vi "WidgetLocation.vi"(6 "error in":errorcluster, 9 "Array in":refnum<class "Array.lvclass">) -> (0 "error out":errorcluster, 3 "Array out":refnum<class "Array.lvclass">, 4 "Bounds":T1, 5 "Location":T2)   [LabVIEW 2014, in "Raspberry Pi Compatible Compiler for LabVIEW.lvlib" / "Array.lvclass"]
uses:
  Array.lvclass
  <vilib>/Utility/miscctls.llb/LVPositionTypeDef.ctl
  <vilib>/Utility/miscctls.llb/LVBoundsTypeDef.ctl
  Control/Control.lvclass
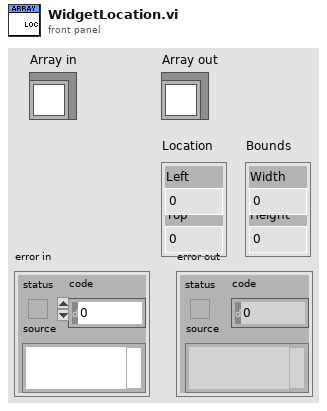
[diagram p1: front panel]
types:
  T1 = typedef "LVBoundsTypeDef.ctl" = cluster{"Width":u32, "Height":u32}
  T2 = typedef "LVPositionTypeDef.ctl" = cluster{"Left":i32, "Top":i32}
  T3 = typedef "LVRectTypeDef.ctl" = cluster{"Left":i16, "Top":i16, "Right":i16, "Bottom":i16}
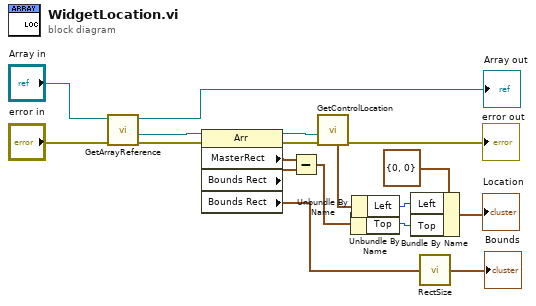
[diagram p0: block diagram]
diagram:
  n1 = call "GetArrayReference.vi"("error in"="error in", "Array in"="Array in") -> ("error out"=w15:errorcluster, "array reference"=w16:refnum<vi>, "Array out"=→"Array out":refnum<class "Array.lvclass">)  [unwired: 7 in]
  n2 = property class="Arr"(reference=w16, error in=w15) -> (reference out=w4:refnum<vi>, error out=w5:errorcluster, "MasterRect"=w14:T3, "Bounds Rect"=w13:T3, "Bounds Rect"=w12:T3)
  n3 = Subtract(x=w14, y=w13) -> (x-y=w8:T3)
  n4 = call "GetControlLocation.vi"("error in"=w5, "Control in"=w4) -> ("error out"=→"error out":errorcluster, "Position"=w2:T2)  [unwired: 5 in, 1 out]
  n5 = Unbundle By Name(w8) -> ("Top"=w9:i16)
  n6 = Unbundle By Name(w2) -> ("Left"=w3:i32)
  n7 = Bundle By Name(cluster=T2 {"Left"=0, "Top"=0} ("Position"), "Left"=w3, "Top"=w9) -> (→"Location":T2)
  n8 = call <vilib>:"RectSize.vi"("rect"=w12) -> ("point"=→"Bounds":cluster{"x":i16, "y":i16})
